vi "WCA_GET_MAG_C.vi"(0 "Cartridge Band":u32=10, 1 "Slave Node in":cluster{"Address":i16, "Serial Number":i8[]}={"Address"=19, "Serial Number"=[16, 71, 55, 76, 1, 8, 0, -15]} {"Serial Number" format="%.0x"; "Address" format="%.0x"}, 2 "ObjHandle in":u32, 5 "POL":u32, 7 "sb":u32=1, 9 "avg":u32=1, 11 "error in (no error)":errorcluster) -> (4 "ObjHandle out":u32=92930112, 8 "GET_MAG_C":dbl=0.35980224609375, 15 "error out":errorcluster)   [LabVIEW 2017]
uses:
  WCA_Global.vi
panel:
  # "Node Address"
  # "Serial Number"
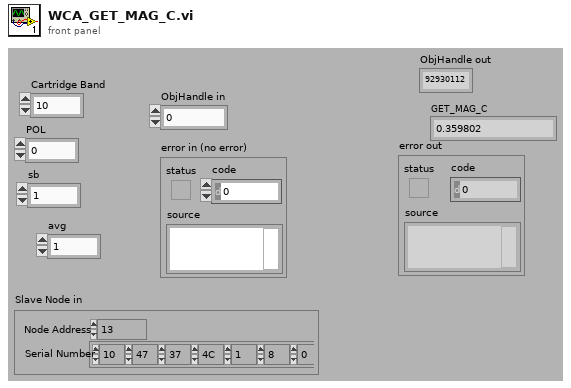
[diagram p1: front panel]
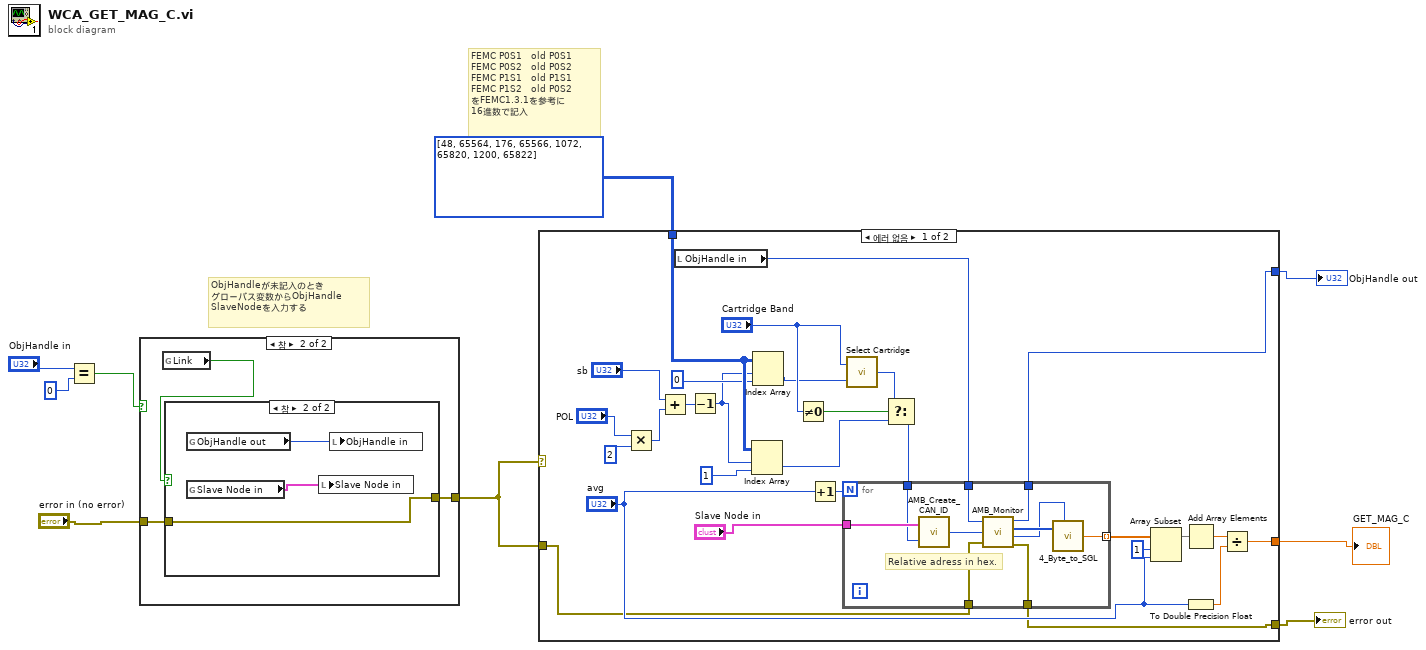
[diagram p0: block diagram]
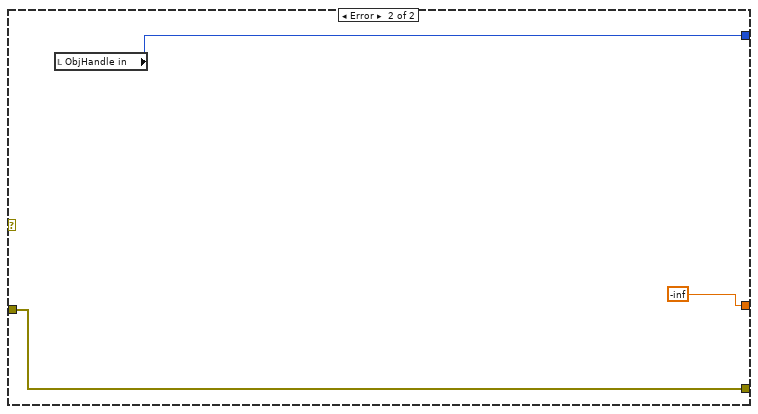
[diagram p2: hidden frame]
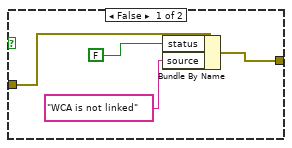
[diagram p4: hidden frame]
diagram:
  # "ObjHandleが未記入のとき\nグローバス変数からObjHandle\nSlaveNodeを入力する"
  # "FEMC P0S1   old P0S1\nFEMC P0S2   old P0S2\nFEMC P1S1   old P1S1\nFEMC P1S2   old P0S2\nをFEMC1.3.1を参考に\n16進数で記入"
  n1 = Equal?(x="ObjHandle in", y=0) -> (x = y?=w7:bool)
  n2 = case shown="참" w7 {
    tunnel: "error in (no error)" -> [w10 w13]
    tunnel: [w10 w12] -> w5
    frame False {
    }
    frame True {
      n3 = global read "WCA_Global.vi" "Link"() -> (w11:bool)
      n4 = case shown="참" w11 {
        tunnel: w13 -> [w17 w18]
        tunnel: [w14 w18] -> w12
        frame False {
          n5 = Bundle By Name(cluster=w17, "status"=FALSE, "source"="WCA is not linked") -> (w14:errorcluster)
        }
        frame True {
          n6 = global read "WCA_Global.vi" "ObjHandle out"() -> (w20:u32)
          n7 = global read "WCA_Global.vi" "Slave Node in"() -> (w19:cluster{"Address":i16, "Serial Number":i8[]})
          n8 = local write "Slave Node in"(w19) -> ()
          n9 = local write "ObjHandle in"(w20) -> ()
        }
      }
    }
  }
  n10 = case shown="에러 없음" w5 {
    tunnel: w5 -> [w32 w61]
    tunnel: [w29 w60] -> w4
    tunnel: [w31 w61] -> w3
    tunnel: i32[][] [[48, 65564], [176, 65566], [1072, 65820], [1200, 65822]] -> [w45 _]
    tunnel: [w35 -inf] -> w1
    frame No Error {
      n11 = Multiply(x="POL", y=2) -> (x*y=w47:u32)
      n12 = Add(x="sb", y=w47) -> (x+y=w46:u32)
      n13 = local read "ObjHandle in"() -> (w30:u32)
      n14 = Decrement(x=w46) -> (x-1=w24:u32)
      n15 = Index Array(array=w45, index (row)=w24, index (col)=1) -> (element=w27:i32)
      n16 = Index Array(array=w45, index (row)=w24, index (col)=0) -> (element=w26:i32)
      n17 = Not Equal To 0?(x="Cartridge Band") -> (x != 0?=w40:bool)
      n18 = Increment(x="avg") -> (x+1=w43:u32)
      n19 = call "Select Cartridge.vi"("Relative Address in"=w26, "Cartridge band"="Cartridge Band") -> ("Relative Address out"=w41:u32)
      n20 = Select(t=w41, s=w40, f=w27) -> (s? t:f=w42:u32)
      n21 = for {
        N: w43 -> [_]
        tunnel: w30 -> [w57]
        tunnel: [w56] -> w29
        tunnel: [w55] -> w31
        tunnel: w32 -> [w54]
        tunnel: "Slave Node in" -> [w53]
        tunnel: [w51] -> w39 mode=indexing
        tunnel: w42 -> [w49]
        # "Relative adress in hex."
        n22 = call "AMB_Create_CAN_ID.vi"("Relative Address in"=w49, "Slave Node in"=w53) -> ("CAN ID out"=w58:u32)
        n23 = call "AMB_Monitor.vi"("ObjHandle in"=w57, "CAN ID in"=w58, "error in"=w54) -> ("ObjHandle out"=w56:u32, "Data Array out"=w52:u8[], "Data Length out"=w50:u8, "error out"=w55:errorcluster)
        n24 = call "4_Byte_to_SGL.vi"("Array of 4 bytes"=w52, "number of valid bytes"=w50) -> ("Number"=w51:sgl)  [unwired: 1 out]
      }
      n25 = Array Subset(array=w39, index=1, length="avg") -> (w37:sgl[])
      n26 = Add Array Elements(numeric array=w37) -> (sum=w36:sgl)
      n27 = To Double Precision Float(number="avg") -> (double precision float=w44:dbl)
      n28 = Divide(x=w36, y=w44) -> (x/y=w35:dbl)
    }
    frame Error {
      n29 = local read "ObjHandle in"() -> (w60:u32)
    }
  }
  "ObjHandle out" <- w4
  "error out" <- w3
  "GET_MAG_C" <- w1
